vi "init.vi"(8 "error in (no error)":errorcluster, 11 "USB IO in":refnum<class "USB IO.lvclass">) -> (0 "error out":errorcluster, 3 "USB IO out":refnum<class "USB IO.lvclass">)   [LabVIEW 2025, in "USB IO.lvclass"]
uses:
  USB IO.lvclass
  USB IO.lvclass/USB IO.ctl
  <vilib>/DAQmx/write.llb/DAQmx Write (Digital 1D Bool NChan 1Samp 1Line).vi
  <vilib>/DAQmx/create/channels.llb/DAQmx Create Channel (DI-Digital Input).vi
  <vilib>/DAQmx/create/channels.llb/DAQmx Create Channel (DO-Digital Output).vi
  <vilib>/DAQmx/miscellaneous.llb/DAQmx Fill In Error Info.vi
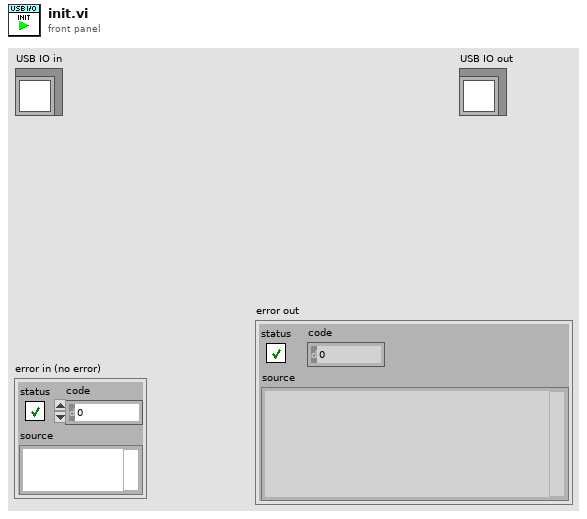
[diagram p1: front panel]
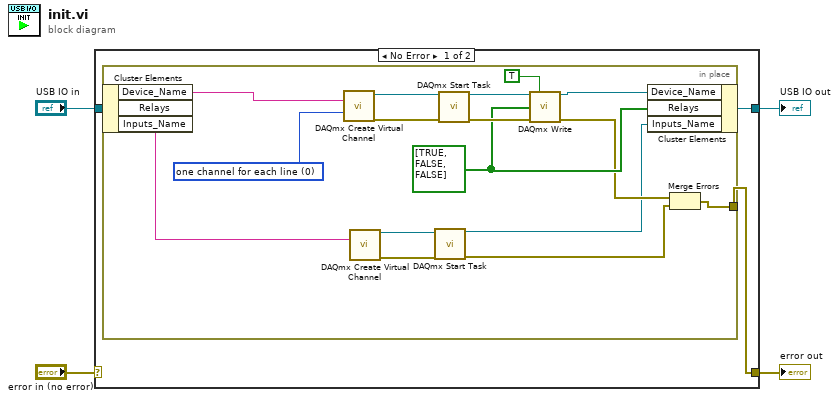
[diagram p0: block diagram]
diagram:
  n1 = case shown="No Error" "error in (no error)" {
    selector: "error in (no error)" -> [_ w25]
    tunnel: [w5 w25] -> w3
    tunnel: [w6 w24] -> w1
    tunnel: "USB IO in" -> [w7 w24]
    frame No Error {
      n2 = in-place {
        in-place-border: [w14] -> w5
        w8 = 0 items=["one channel for each line", "one channel for all lines"] ("line grouping")
        w16 = bool[] [TRUE, FALSE, FALSE] ("data")
        n3 = in-place-cluster #1(w7) -> ("Device_Name"=w23:string, "Inputs_Name"=w15:string)  [unwired: 1 out]
        n4 = call-poly <vilib>:"DAQmx Create Virtual Channel.vi"("lines"=w23, "line grouping"=w8) -> ("task out"=w22:refnum<k21>, "error out"=w21:errorcluster)  [unwired: 12 in]
        n5 = call-poly <vilib>:"DAQmx Create Virtual Channel.vi"("lines"=w15) -> ("task out"=w12:refnum<k21>, "error out"=w11:errorcluster)  [unwired: 13 in]
        n6 = call <vilib>:"DAQmx Start Task.vi"("task/channels in"=w12, "error in"=w11) -> ("task out"=w10:refnum<k21>, "error out"=w9:errorcluster)  [unwired: 12 in]
        n7 = call <vilib>:"DAQmx Start Task.vi"("task/channels in"=w22, "error in"=w21) -> ("task out"=w20:refnum<k21>, "error out"=w19:errorcluster)  [unwired: 12 in]
        n8 = call-poly <vilib>:"DAQmx Write.vi"("task/channels in"=w20, "auto start"=TRUE, "data"=w16, "error in"=w19) -> ("task out"=w17:refnum<k21>, "error out"=w13:errorcluster)  [unwired: 9 in, 1 out]
        n9 = in-place-cluster #1("Device_Name"=w17, "Relays"=w16, "Inputs_Name"=w10) -> (w6:refnum<class "USB IO.lvclass">)
        n10 = Merge Errors(w13, w9) -> (w14:errorcluster)
      }
    }
    frame Error {
    }
  }
  "error out" <- w3
  "USB IO out" <- w1
